vi "read control value - polymorphic.vi"   [LabVIEW 2024, in "controls manager.lvlib"]
uses:
  controls manager.lvlib
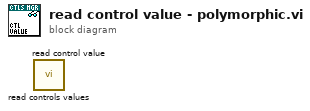
[diagram p0: block diagram]
diagram:
  n1 = call "read controls values.vi"() -> ()  [unwired: 10 in, 2 out]
  n2 = call "read control value.vi"() -> ()  [unwired: 10 in, 2 out]
